vi "Main IU.vi"() -> ()   [LabVIEW 2018]
uses:
  <vilib>/Analysis/baseanly.llb/Mean (DBL).vi
  <vilib>/Utility/file.llb/Read Delimited Spreadsheet (DBL).vi
  <vilib>/Analysis/NI_AALBase.lvlib
panel:
  out "Actual Y":dbl
  out "ActualX":dbl
  in  "Escriba el tiempo para ejecutar\ntrayectoria suave":dbl
  in  "Setpoint 2":dbl min=-2.5 max=2.5 step=0.1
  in  "Setpoint 1":dbl min=-1.5 max=1.5 step=0.1
  in  "Homing":bool
  out "EsfuerzoSat 2":dbl(graph)
  out "SetpointVsSalida 2":cluster{"Double":dbl, "Output":dbl}(graph)
  out "Posicion actual":dbl(graph)
  out "SetpointVsSalida":cluster{"Double":dbl, "Output":dbl}(graph)
  out "Saving Data":bool
  in  "Record Button":bool
  in  "Filename":path=path "test.lvm"
  out "Motor1":waveform(dbl)[](graph)
  in  "Paro Emergencia:\nUI y RT":bool
  in  "Stop UI":bool
  # "s"
  # "Esta automáticamente se ejecutará"
  # "rad/s^2"
  # "rad/s^2"
  # "rad"
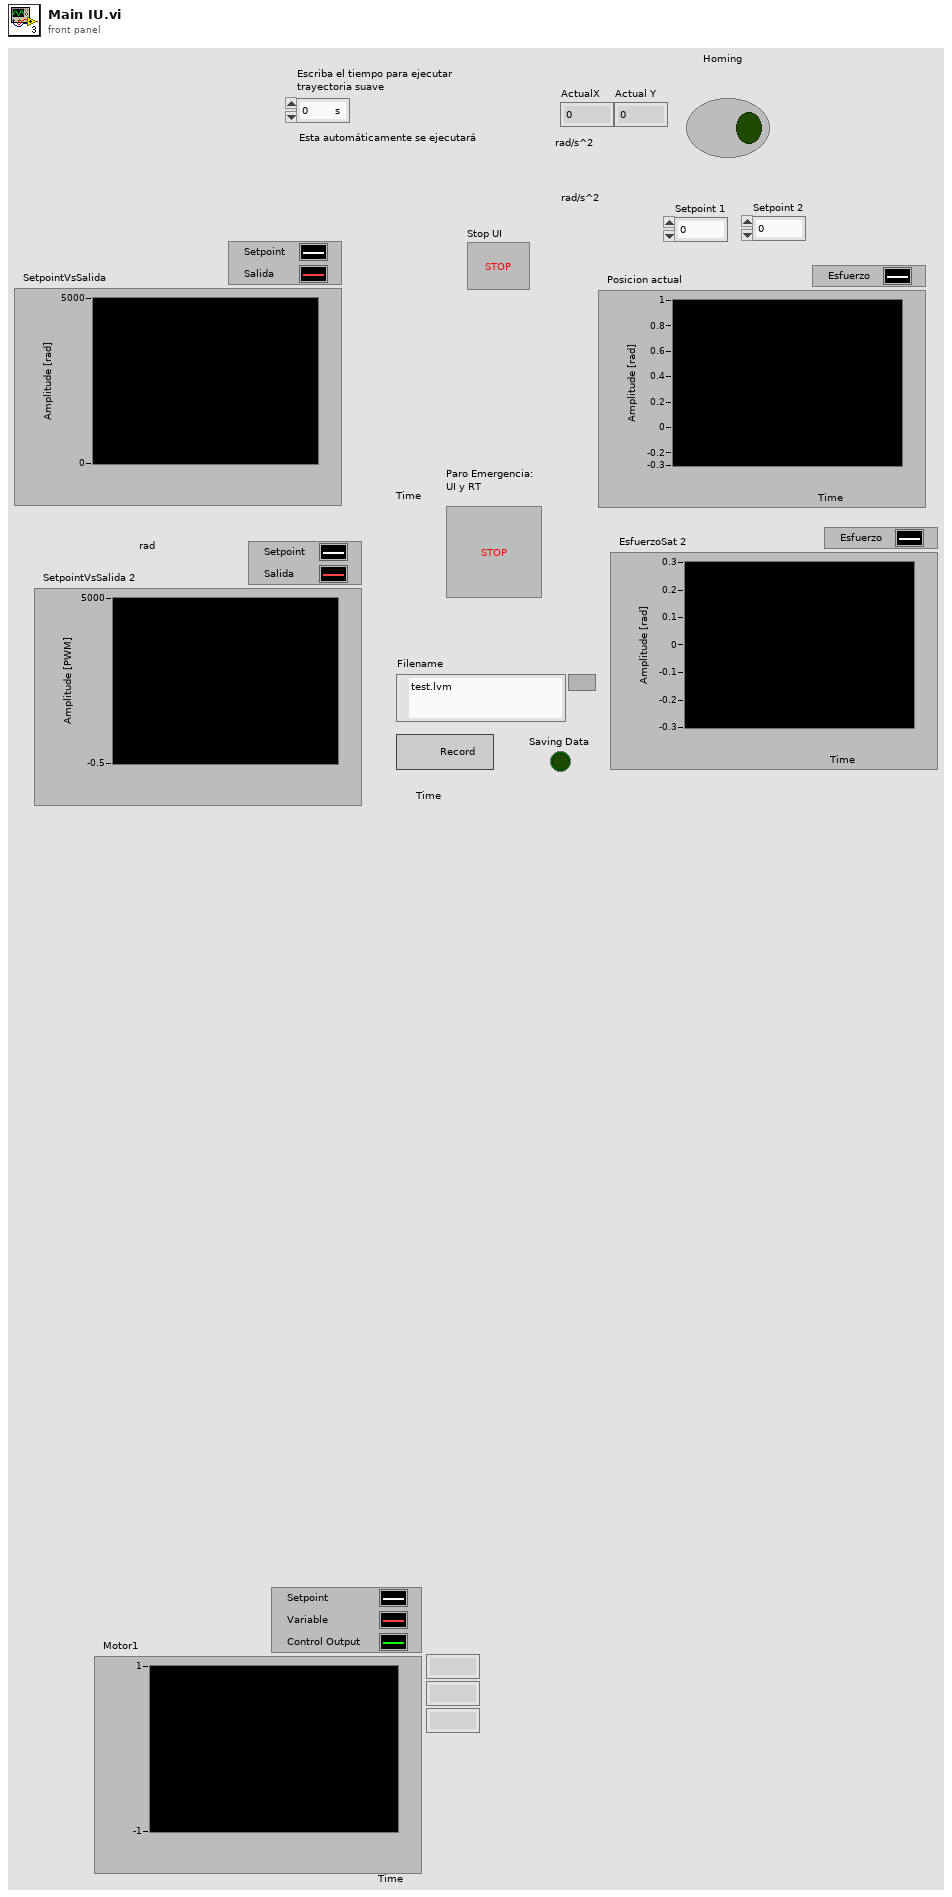
[diagram p1: front panel]
types:
  T1 = cluster{"Double":dbl, "dbl Scaled Value":dbl, "Output":dbl, "seconds since 1Jan1904":timestamp, dbl, dbl, dbl}
  T2 = cluster{"writer name":string, "Variant":variant, "Variant":variant}
  T3 = cluster{"Double":dbl, "dbl Scaled Value":dbl, "Output":dbl, "seconds since 1Jan1904":timestamp, dbl, dbl, dbl}[]
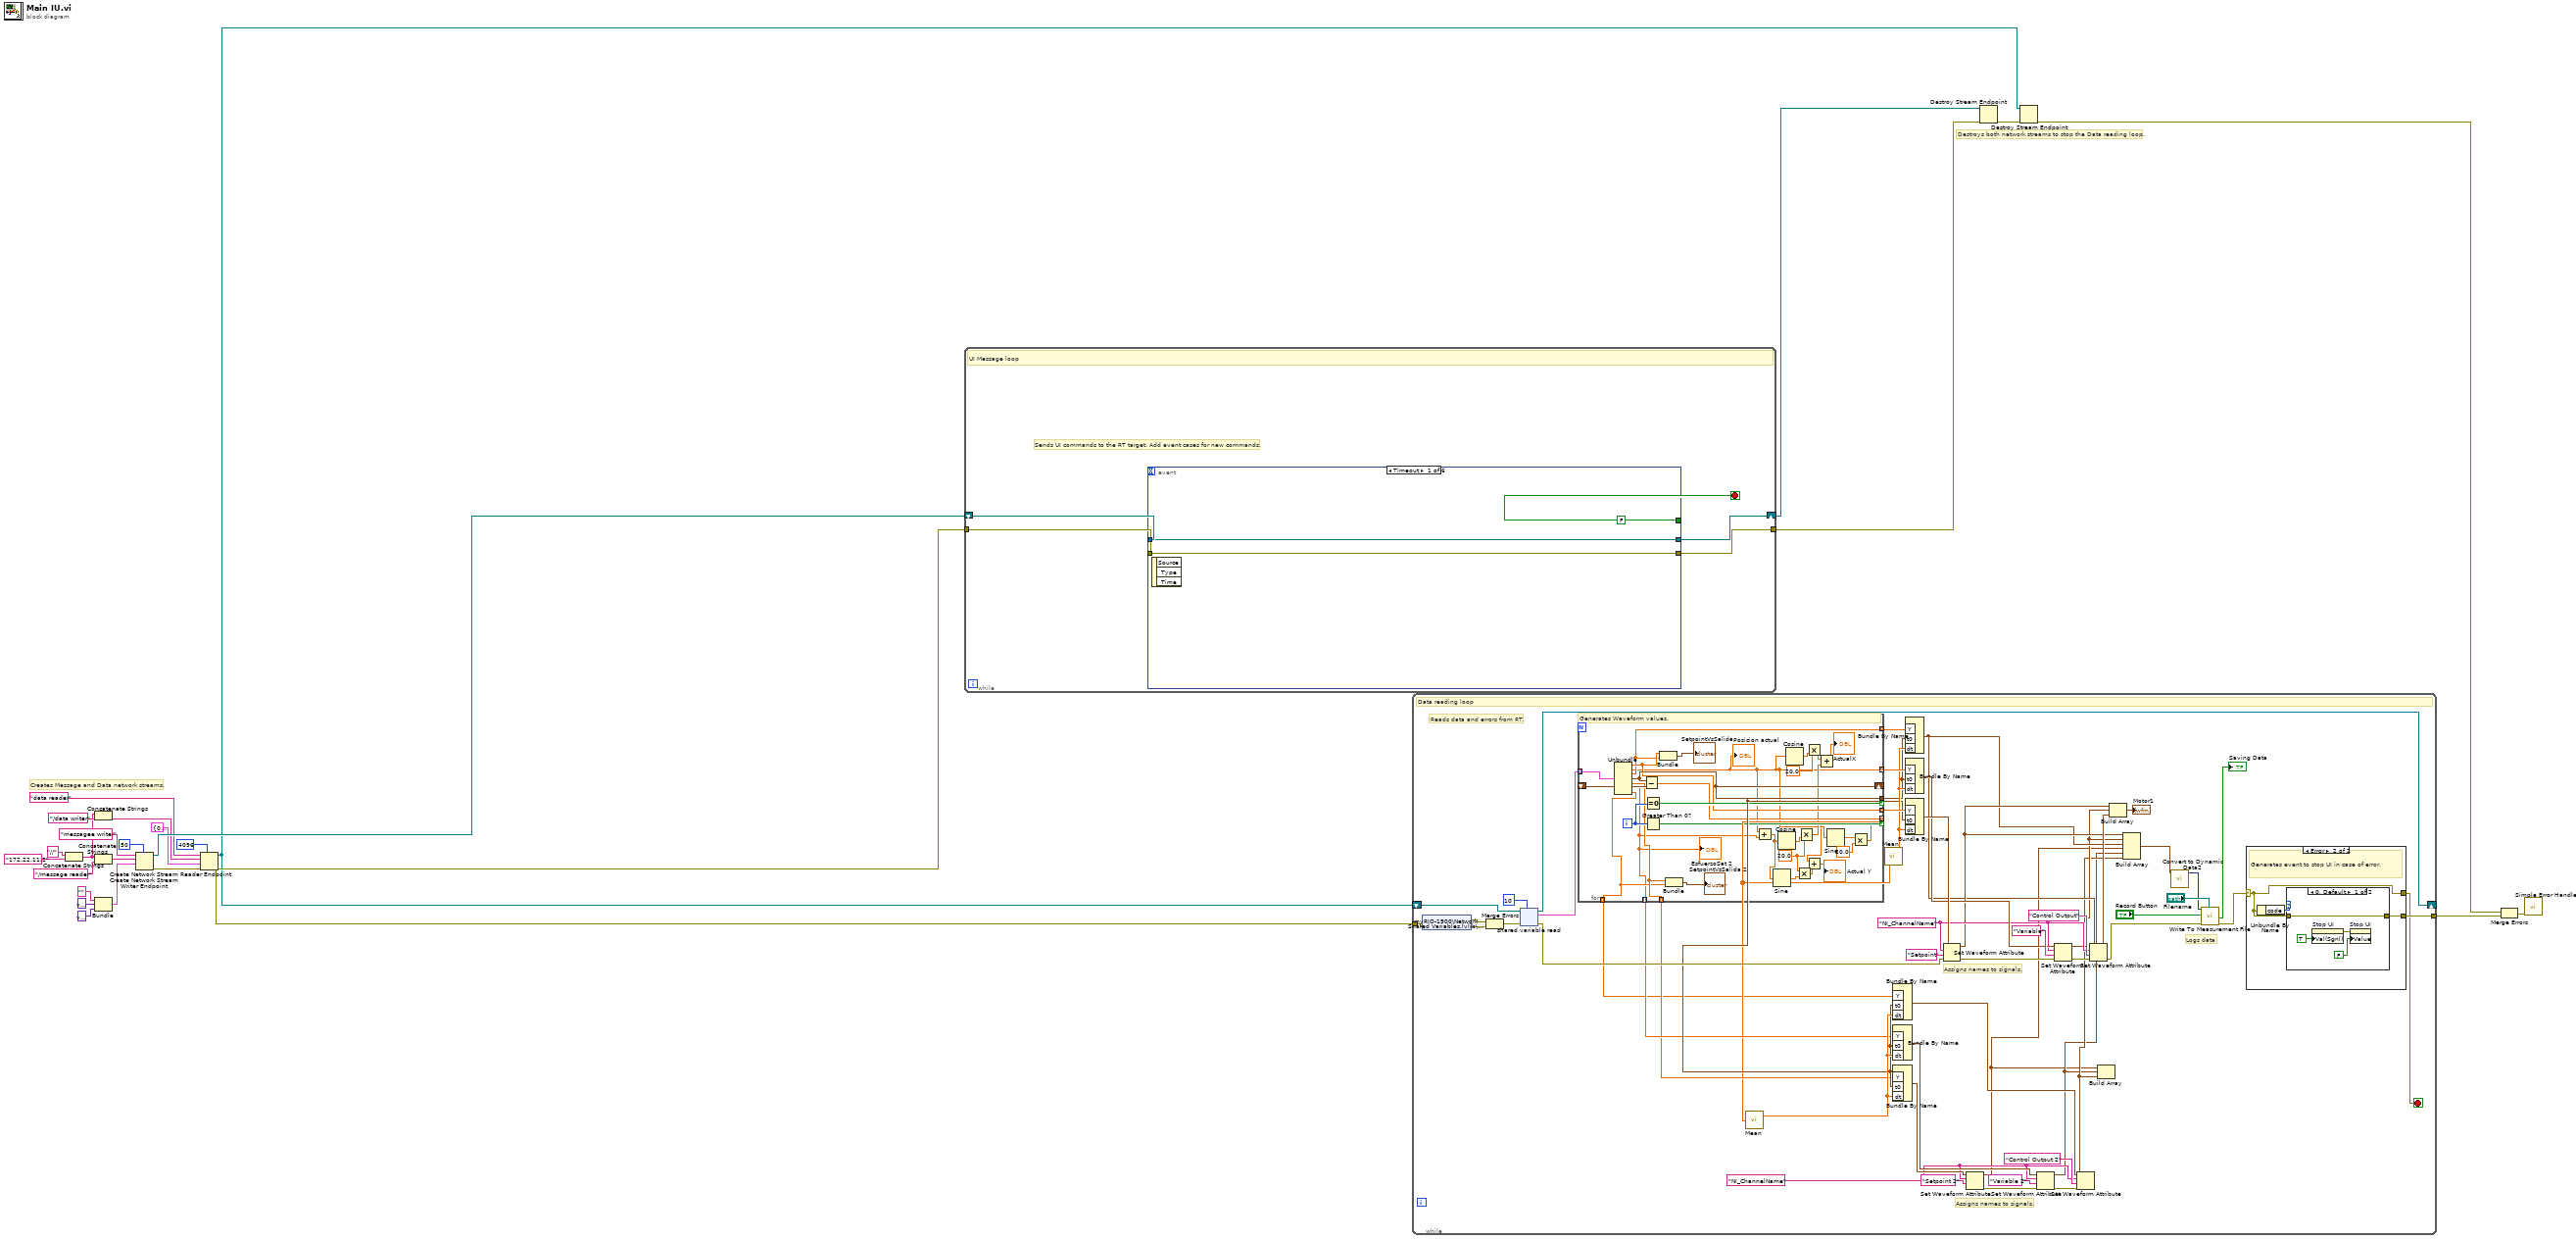
[diagram p0: block diagram]
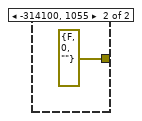
[diagram p3: hidden frame]
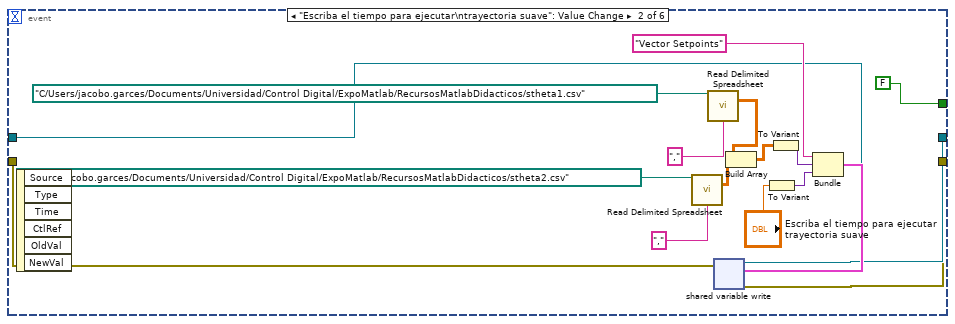
[diagram p4: hidden frame]
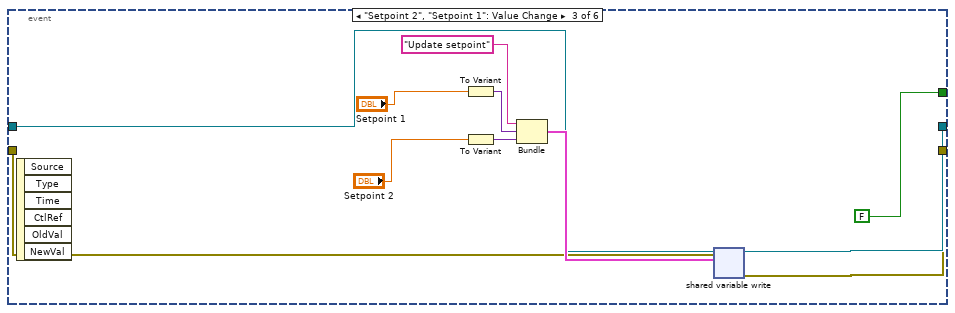
[diagram p5: hidden frame]
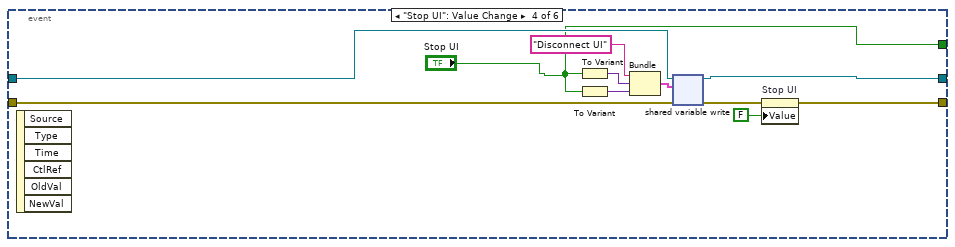
[diagram p6: hidden frame]
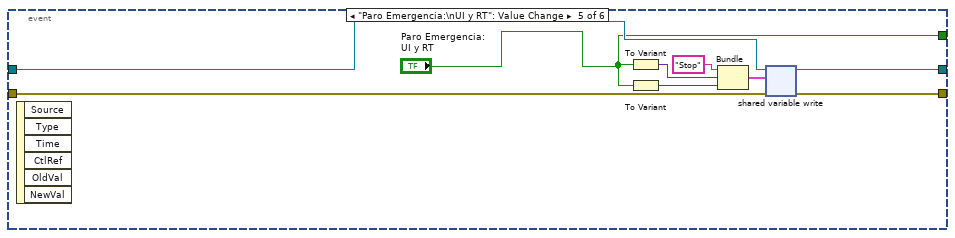
[diagram p7: hidden frame]
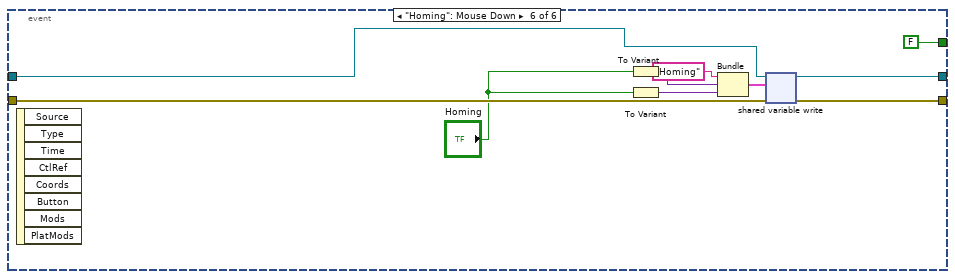
[diagram p8: hidden frame]
diagram:
  # "Destroys both network streams to stop the Data reading loop."
  # "Creates Message and Data network streams."
  n1 = Concatenate Strings("//", "172.22.11.2" ("myRIO IP")) -> (w2:string)
  n2 = Bundle("", variant, variant) -> (w26:cluster{string, variant, variant})  [unwired: 1 in]
  n3 = Concatenate Strings(w2, "/data writer") -> (w17:string)
  n4 = Concatenate Strings(w2, "/message reader") -> (w3:string)
  n5 = Create Network Stream Writer Endpoint(7:50 ("writer buffer size"), 9:w26, 10:w3, 11:"messagee writer" ("writer name")) -> (0:w14:errorcluster, 3:w20:refnum<k21>)  [unwired: 3 in]
  n6 = Create Network Stream Reader Endpoint(7:4096 ("reader buffer size"), 8:w14, 9:T1 {"Double"=0.0, "dbl Scaled Value"=0.0, "Output"=0.0, "seconds since 1Jan1904"=timestamp(0 s since 1904-01-01), 0.0, 0.0, 0.0} ("Data"), 10:w17, 11:"data reader" ("reader name")) -> (0:w13:errorcluster, 3:w6:refnum<k21>)  [unwired: 2 in]
  n7 = while {
    tunnel: w13 -> [w27]
    shift-right: [w31] -> w8
    shift-left: w20 -> [w28]
    tunnel: [w30] -> w9
    stop <- w29 stop-if-true
    # "Sends UI commands to the RT target. Add event cases for new commands."
    # "UI Message loop"
    n8 = event shown="[0] Timeout" {
      selector: _ -> [_ _ _ _ _ _]
      dyn-events: _ -> [_ _ _ _ _ _]
      timeout: _ -> [_ _ _ _ _ _]
      tunnel: [w33 w46 w57 w70 w78 w88] -> w31
      tunnel: [w32 w45 w56 w67 w79 w89] -> w30
      tunnel: [FALSE ("Stop UI and RT") FALSE ("Stop UI and RT") FALSE ("Stop UI and RT") "Stop UI" "Paro Emergencia:\nUI y RT" FALSE] -> w29
      tunnel: w28 -> [w33 w44 w55 w64 w76 w86]
      tunnel: w27 -> [w32 w43 w54 w65 w75 w85]
      event Timeout {
        n9 = event-data() -> ()  [unwired: 1 in, 3 out]
      }
      event "Escriba el tiempo para ejecutar\ntrayectoria suave": Value Change {
        n10 = event-data() -> ()  [unwired: 1 in, 6 out]
        n11 = call-poly <vilib>:"Read Delimited Spreadsheet.vi"("file path (dialog if empty)"=path "C:/Users/jacobo.garces/Documents/Universidad/Control Digital/ExpoMatlab/RecursosMatlabDidacticos/stheta2.csv", "delimiter (\\t)"="," ("delimiter (\\t)")) -> ("all rows"=w38:dbl[][])  [unwired: 8 in, 5 out]
        n12 = call-poly <vilib>:"Read Delimited Spreadsheet.vi"("file path (dialog if empty)"=path "C:/Users/jacobo.garces/Documents/Universidad/Control Digital/ExpoMatlab/RecursosMatlabDidacticos/stheta1.csv", "delimiter (\\t)"="," ("delimiter (\\t)")) -> ("all rows"=w37:dbl[][])  [unwired: 8 in, 5 out]
        n13 = Build Array(w37, w38) -> (w36:dbl[][][])
        n14 = To Variant(anything="Escriba el tiempo para ejecutar\ntrayectoria suave") -> (Variant=w49:variant)
        n15 = To Variant(anything=w36) -> (Variant=w47:variant)
        n16 = Bundle("writer name"="Vector Setpoints", "Variant"=w47, "Variant"=w49) -> (w48:T2)  [unwired: 1 in]
        n17 = shared-variable-write(w44, w43, w48) -> (w46:refnum<k21>, w45:errorcluster)  [unwired: 1 in, 1 out]
      }
      event "Setpoint 2", "Setpoint 1": Value Change {
        n18 = event-data() -> ()  [unwired: 1 in, 6 out]
        n19 = To Variant(anything="Setpoint 1") -> (Variant=w58:variant)
        n20 = To Variant(anything="Setpoint 2") -> (Variant=w60:variant)
        n21 = Bundle("writer name"="Update setpoint", "Variant"=w58, "Variant"=w60) -> (w59:T2)  [unwired: 1 in]
        n22 = shared-variable-write(w55, w54, w59) -> (w57:refnum<k21>, w56:errorcluster)  [unwired: 1 in, 1 out]
      }
      event "Stop UI": Value Change {
        n23 = event-data() -> ()  [unwired: 1 in, 6 out]
        n24 = To Variant(anything="Stop UI") -> (Variant=w73:variant)
        n25 = To Variant(anything="Stop UI") -> (Variant=w66:variant)
        n26 = Bundle("writer name"="Disconnect UI", "Variant"=w73, "Variant"=w66) -> (w72:T2)  [unwired: 1 in]
        n27 = shared-variable-write(w64, w65, w72) -> (w70:refnum<k21>, w68:errorcluster)  [unwired: 1 in, 1 out]
        n28 = property on="Stop UI" class="Bool (strict)"(error in=w68, "Value"=FALSE ("Stop UI and RT")) -> (error out=w67:errorcluster)  [unwired: 1 in, 1 out]
      }
      event "Paro Emergencia:\nUI y RT": Value Change {
        n29 = event-data() -> ()  [unwired: 1 in, 6 out]
        n30 = To Variant(anything="Paro Emergencia:\nUI y RT") -> (Variant=w82:variant)
        n31 = To Variant(anything="Paro Emergencia:\nUI y RT") -> (Variant=w77:variant)
        n32 = Bundle("writer name"="Stop", "Variant"=w82, "Variant"=w77) -> (w81:T2)  [unwired: 1 in]
        n33 = shared-variable-write(w76, w75, w81) -> (w78:refnum<k21>, w79:errorcluster)  [unwired: 1 in, 1 out]
      }
      event "Homing": Mouse Down {
        n34 = event-data() -> ()  [unwired: 1 in, 8 out]
        n35 = To Variant(anything="Homing") -> (Variant=w92:variant)
        n36 = To Variant(anything="Homing") -> (Variant=w87:variant)
        n37 = Bundle("writer name"="Homing", "Variant"=w92, "Variant"=w87) -> (w91:T2)  [unwired: 1 in]
        n38 = shared-variable-write(w86, w85, w91) -> (w88:refnum<k21>, w89:errorcluster)  [unwired: 1 in, 1 out]
      }
    }
  }
  n39 = while {
    tunnel: w13 -> [w120]
    shift-right: [w130] -> _
    shift-left: w6 -> [w145]
    tunnel: [w119] -> w10
    stop <- w118 stop-if-true
    w107 = "NI_ChannelName" ("name")
    w124 = "NI_ChannelName" ("name")
    # "Assigns names to signals."
    # "Logs data"
    # "Assigns names to signals."
    # "Reads data and errors from RT."
    # "Data reading loop"
    n40 = shared-variable "myRIO-1900\\Network Shared Variables.lvlib\\error IO"(error in=w120) -> (w123:errorcluster, error out=w122:errorcluster)
    n41 = Merge Errors(w123, w122) -> (w121:errorcluster)
    n42 = shared-variable-read(w145, w121, 10 ("# elements")) -> (w130:refnum<k21>, w135:errorcluster, w143:T3)  [unwired: 1 in, 1 out]
    n43 = for {
      tunnel: w143 -> [w183] mode=indexing
      tunnel: [w176] -> w142 mode=indexing
      tunnel: [w159] -> w141 mode=indexing
      tunnel: [w175] -> w117 mode=indexing
      tunnel: [w181] -> w106 if=w182
      shift-right: [w181] -> _
      shift-left: _ -> [w180]
      tunnel: [w179] -> w103 mode=indexing if=w177
      tunnel: [w171] -> w102 mode=indexing
      tunnel: [w167] -> w105 mode=indexing
      tunnel: [w172] -> w104 mode=indexing
      i -> [w178]
      w161 = 20.0 ("x")
      # "Generates Waveform values."
      n44 = Unbundle(w183) -> ("Double"=w176:dbl, "dbl Scaled Value"=w159:dbl, "Output"=w175:dbl, "seconds since 1Jan1904"=w181:timestamp, w172:dbl, w167:dbl, w171:dbl)
      "Posicion actual" <- w159
      "EsfuerzoSat 2" <- w167
      n45 = Subtract(x=w181, y=w180) -> (x-y=w179:dbl)
      n46 = Equal To 0?(x=w178) -> (x = 0?=w182:bool)
      n47 = Greater Than 0?(x=w178) -> (x > 0?=w177:bool)
      n48 = Bundle("Double"=w176, "Output"=w175) -> (→"SetpointVsSalida":cluster{"Double":dbl, "Output":dbl})  [unwired: 1 in]
      n49 = Bundle(w172, w171) -> (→"SetpointVsSalida 2":cluster{dbl, dbl})  [unwired: 1 in]
      n50 = Add(x=w159, y=w167) -> (x+y=w163:dbl)
      n51 = Sine(x=w163) -> (sin(x)=w162:dbl)
      n52 = Cosine(x=w163) -> (cos(x)=w168:dbl)
      n53 = Cosine(x=w159) -> (cos(x)=w170:dbl)
      n54 = Multiply(x=w161, y=w162) -> (x*y=w160:dbl)
      n55 = Multiply(x=w161, y=w168) -> (x*y=w165:dbl)
      n56 = Multiply(x=20.0, y=w170) -> (x*y=w166:dbl)
      n57 = Add(x=w166, y=w165) -> (x+y=→"ActualX":dbl)
      n58 = Sine(x=w159) -> (sin(x)=w158:dbl)
      n59 = Multiply(x=w158, y=20.0 ("x")) -> (x*y=w155:dbl)
      n60 = Add(x=w155, y=w160) -> (x+y=→"Actual Y":dbl)
    }
    n61 = call-poly <vilib>:"Mean.vi"("X"=w103) -> ("mean"=w116:dbl)  [unwired: 1 out]
    n62 = call-poly <vilib>:"Mean.vi"("X"=w103) -> ("mean"=w140:dbl)  [unwired: 1 out]
    n63 = Bundle By Name("Y"=w102, "t0"=w106, "dt"=w116) -> (w108:waveform(dbl))  [unwired: 1 in]
    n64 = Bundle By Name("Y"=w105, "t0"=w106, "dt"=w116) -> (w109:waveform(dbl))  [unwired: 1 in]
    n65 = Bundle By Name("Y"=w104, "t0"=w106, "dt"=w116) -> (w115:waveform(dbl))  [unwired: 1 in]
    n66 = Bundle By Name("Y"=w117, "t0"=w106, "dt"=w140) -> (w98:waveform(dbl))  [unwired: 1 in]
    n67 = Bundle By Name("Y"=w141, "t0"=w106, "dt"=w140) -> (w132:waveform(dbl))  [unwired: 1 in]
    n68 = Bundle By Name("Y"=w142, "t0"=w106, "dt"=w140) -> (w139:waveform(dbl))  [unwired: 1 in]
    n69 = Set Waveform Attribute(4:w135, 5:"Setpoint" ("name"), 6:w124, 7:w139) -> (0:w134:errorcluster, 3:w99:waveform(dbl))  [unwired: 1 out]
    n70 = Set Waveform Attribute(5:"Setpoint 2" ("name"), 6:w107, 7:w115) -> (0:w111:errorcluster, 3:w94:waveform(dbl))  [unwired: 1 in, 1 out]
    n71 = Set Waveform Attribute(4:w111, 5:"Variable 2" ("name"), 6:w107, 7:w109) -> (0:w110:errorcluster, 3:w95:waveform(dbl))  [unwired: 1 out]
    n72 = Set Waveform Attribute(4:w134, 5:"Variable" ("name"), 6:w124, 7:w132) -> (0:w133:errorcluster, 3:w97:waveform(dbl))  [unwired: 1 out]
    n73 = Set Waveform Attribute(4:w110, 5:"Control Output 2" ("name"), 6:w107, 7:w108) -> (3:w96:waveform(dbl))  [unwired: 2 out]
    n74 = Set Waveform Attribute(4:w133, 5:"Control Output" ("name"), 6:w124, 7:w98) -> (0:w129:errorcluster, 3:w131:waveform(dbl))  [unwired: 1 out]
    n75 = Build Array(w94, w95, w96) -> ()  [unwired: 1 out]
    n76 = Build Array(w99, w97, w131) -> (→"Motor1":waveform(dbl)[])
    n77 = Build Array(w99, w97, w98, w94, w95, w96) -> (w93:waveform(dbl)[])
    n78 = call "Convert to Dynamic Data2"("Array of Waveforms"=w93) -> ("Dynamic Data Type"=w100:dynamicdata)  [unwired: 3 in]
    n79 = call "Write To Measurement File"("Signals"=w100, "Enable"="Record Button", "error in (no error)"=w129, "Filename"="Filename") -> ("Saving Data"=→"Saving Data":bool, "error out"=w125:errorcluster)  [unwired: 13 in, 1 out]
    n80 = case shown="Error" w125 {
      selector: w125 -> [w146 w147]
      tunnel: [w146 w148] -> w119
      tunnel: [w146 w147] -> w118
      frame No Error {
        # "No action required."
      }
      frame Error {
        # "Generates event to stop UI in case of error."
        n81 = Unbundle By Name(w147) -> ("code"=w149:i32)
        n82 = case shown="0, Default" w149 {
          tunnel: [w152 errorcluster {"status"=FALSE, "code"=0, "source"=""} ("error IO")] -> w148
          tunnel: w147 -> [w152 _]
          frame 0, Default {
            n83 = property on="Stop UI" class="Bool (strict)"("Val(Sgnl)"=TRUE ("Stop UI and RT")) -> (error out=w151:errorcluster)  [unwired: 2 in, 1 out]
            n84 = property on="Stop UI" class="Bool (strict)"(error in=w151, "Value"=FALSE ("Stop UI")) -> ()  [unwired: 1 in, 2 out]
          }
          frame -314100, 1055 {
          }
        }
      }
    }
  }
  n85 = Destroy Stream Endpoint(8:w9, 11:w8) -> (0:w7:errorcluster)
  n86 = Destroy Stream Endpoint(8:w7, 11:w6) -> (0:w5:errorcluster)
  n87 = Merge Errors(w5, w10) -> (w11:errorcluster)
  n88 = call <vilib>:"Simple Error Handler.vi"("error in (no error)"=w11) -> ()  [unwired: 4 in, 5 out]
